vi "StoreOperateMode.vi"(8 "error in (no error)":errorcluster, 9 "eOperateMode":u16(ring) items=["Continuous", "Burst"], 11 "ClassIn":refnum<class "NISTFGenPluginsBase.lvclass">) -> (0 "error out":errorcluster, 3 "ClassOut":refnum<class "NISTFGenPluginsBase.lvclass">)   [LabVIEW 2014, in "FGenPlugins.lvlib" / "NISTFGenPluginsBase.lvclass"]
uses:
  NISTFGenPluginsBase.lvclass
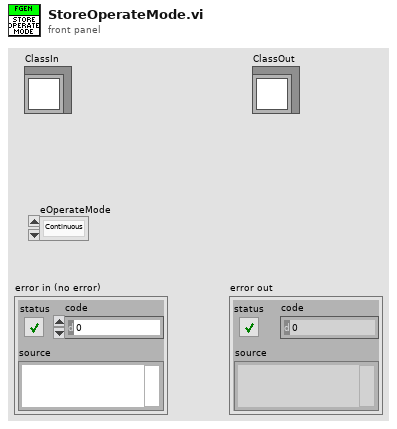
[diagram p1: front panel]
types:
  T1 = typedef "FGenPlugins.lvlib/NISTFGenPluginsBase.lvclass/ChannelParamElement.ctl" = cluster{"sName":string, "eOperateMode":u16, "bEnabled":bool, "eOutputMode":u16, "iIndex":i32, "iNameBufferSize":i32, "fGain":dbl}
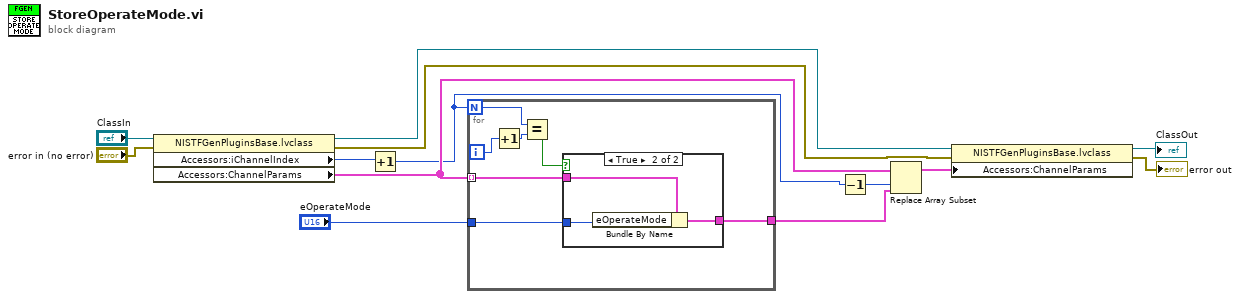
[diagram p0: block diagram]
diagram:
  n1 = property class="NISTFGenPluginsBase.lvclass"(reference="ClassIn", error in="error in (no error)") -> (reference out=w6:refnum<class "NISTFGenPluginsBase.lvclass">, error out=w5:errorcluster, "Accessors:iChannelIndex"=w3:i32, "Accessors:ChannelParams"=w4:T1[])
  n2 = Increment(x=w3) -> (x+1=w2:i32)
  n3 = for {
    N: w2 -> [w14]
    tunnel: w4 -> [w19] mode=indexing
    tunnel: "eOperateMode" -> [w18]
    tunnel: [w17] -> w11
    i -> [w16]
    n4 = Increment(x=w16) -> (x+1=w15:i32)
    n5 = Equal?(x=w14, y=w15) -> (x = y?=w20:bool)
    n6 = case shown="True" w20 {
      tunnel: w19 -> [w21 w24]
      tunnel: w18 -> [_ w23]
      tunnel: [w21 w22] -> w17
      frame False {
      }
      frame True {
        n7 = Bundle By Name(cluster=w24, "eOperateMode"=w23) -> (w22:T1)
      }
    }
  }
  n8 = Decrement(x=w2) -> (x-1=w1:i32)
  n9 = Replace Array Subset(array=w4, new element=w11, index=w1) -> (w10:T1[])
  n10 = property class="NISTFGenPluginsBase.lvclass"(reference=w6, error in=w5, "Accessors:ChannelParams"=w10) -> (reference out=→"ClassOut":refnum<class "NISTFGenPluginsBase.lvclass">, error out=→"error out":errorcluster)
